vi "arduinoSetValve.vi"(0 "command":u8 max=63 step=1) -> ()   [LabVIEW 2012]
uses:
  GlobalArduino.vi
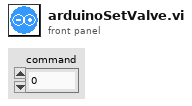
[diagram p1: front panel]
types:
  T1 = typedef "Semaphore RefNum" = refnum<k1>
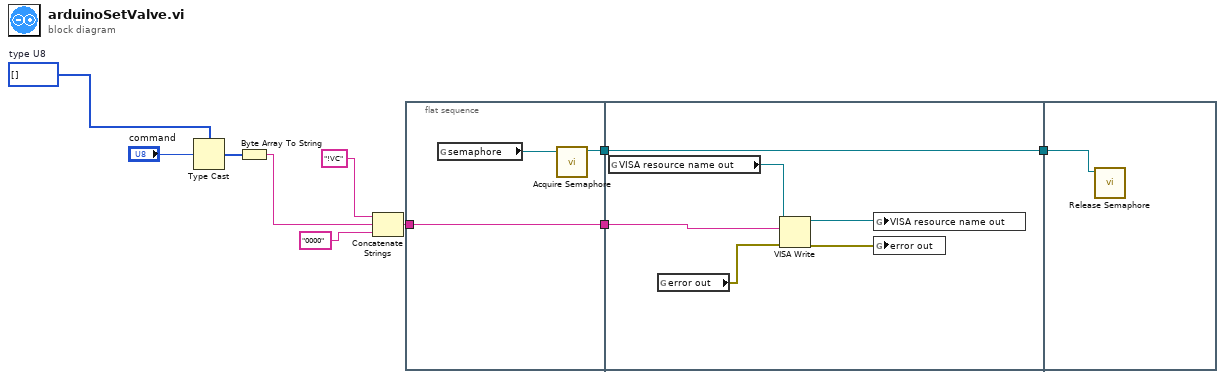
[diagram p0: block diagram]
diagram:
  w9 = u8[] []  # type U8
  n1 = Type Cast(type=w9, x="command") -> (*(type *) &x=w8:u8[])
  n2 = Byte Array To String(unsigned byte array=w8) -> (string=w5:string)
  n3 = Concatenate Strings("!VC" ("string"), w5, "0000" ("string")) -> (w6:string)
  n4 = flat-sequence {
    tunnel: w6 -> [w13]
    tunnel: [w13] -> w3
    tunnel: [w11] -> w2
    tunnel: w3 -> [w19]
    tunnel: w2 -> [w14]
    tunnel: [w14] -> w1
    tunnel: w1 -> [w20]
    frame #0 {
      n5 = global read "GlobalArduino.vi" "semaphore"() -> (w12:T1)
      n6 = call <vilib>:"Acquire Semaphore.vi"("semaphore"=w12) -> ("semaphore out"=w11:T1)  [unwired: 4 in, 2 out]
    }
    frame #1 {
      n7 = global read "GlobalArduino.vi" "VISA resource name out"() -> (w18:refnum<visa-resource-name>)
      n8 = global read "GlobalArduino.vi" "error out"() -> (w16:errorcluster)
      n9 = VISA Write(VISA resource name=w18, write buffer=w19, error in (no error)=w16) -> (VISA resource name out=w17:refnum<visa-resource-name>, error out=w15:errorcluster)  [unwired: 1 out]
      n10 = global write "GlobalArduino.vi" "VISA resource name out"(w17) -> ()
      n11 = global write "GlobalArduino.vi" "error out"(w15) -> ()
    }
    frame #2 {
      n12 = call <vilib>:"Release Semaphore.vi"("semaphore"=w20) -> ()  [unwired: 5 in, 2 out]
    }
  }
